vi "5x Lesen System ini.vi"(8 "Fehler (Eingang, kein Fehler)":errorcluster, 9 "Factorysettings":path, 11 "appended path":path) -> (0 "Fehler (Ausgang)":errorcluster, 2 "Sys Log Level":i32, 4 "Datenfluss (out)":bool)   [LabVIEW 2020, in "Konfig-Dateien.lvlib"]
uses:
  Konfig-Dateien.lvlib
  SysLog/SysLog Interface cRIO.ctl
  <vilib>/Utility/config.llb/Read Key (I32).vi
  <vilib>/Utility/config.llb/NI_LVConfig.lvlib
  SysLog/SysLog_cRIO.lvlib
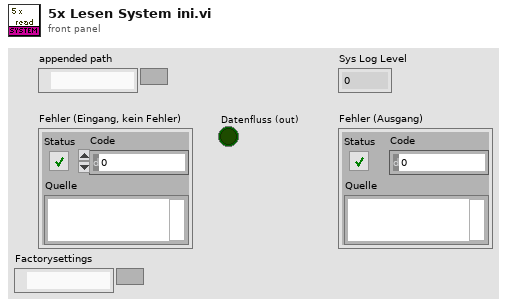
[diagram p1: front panel]
types:
  T1 = typedef "NI_LVConfig.lvlib/Config Data RefNum.ctl" = refnum<k1>
  T2 = typedef "SysLog_cRIO.lvlib/SysLog Interface cRIO.ctl" = cluster{"FehlermeldungsCode":i32, "ErfolgsmeldungsCode":i32, "ParameterListenString":string, "intern":bool}
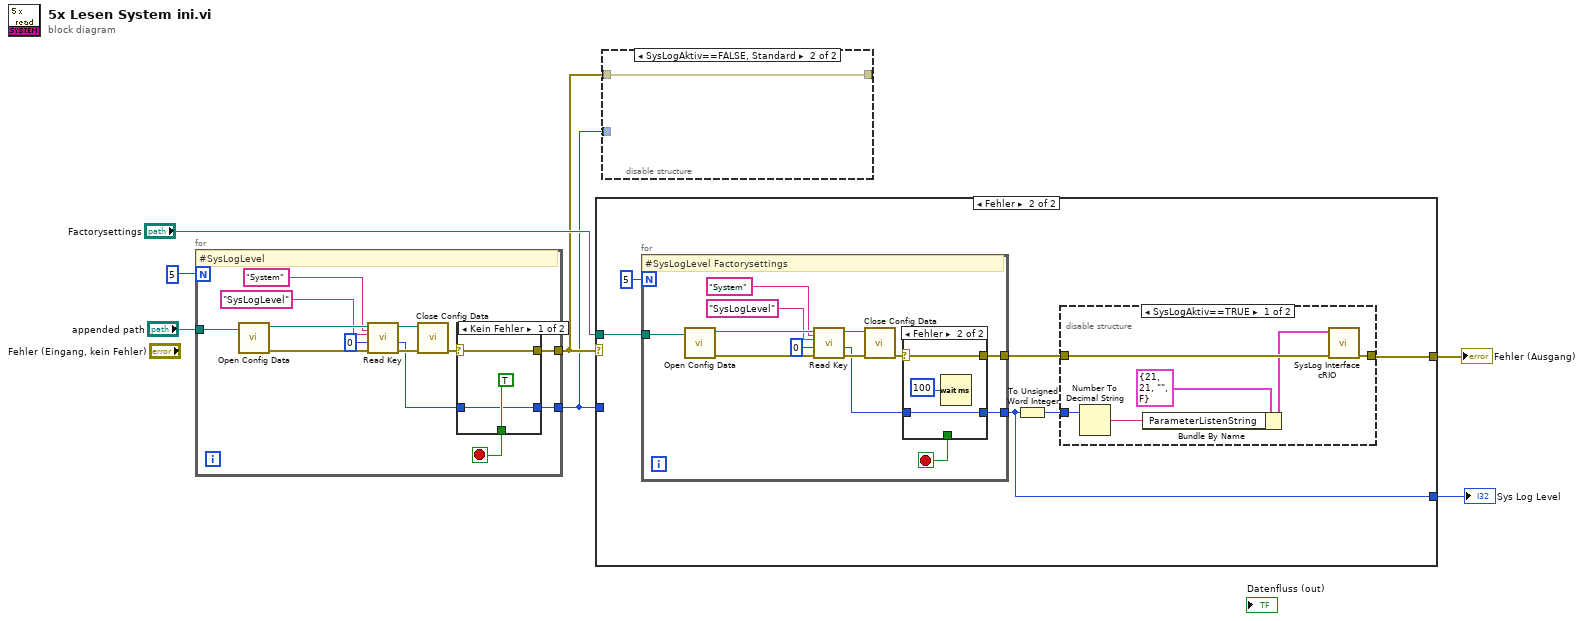
[diagram p0: block diagram]
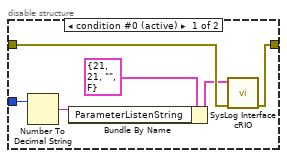
[diagram p2: hidden frame]
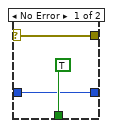
[diagram p5: hidden frame]
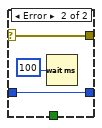
[diagram p6: hidden frame]
diagram:
  n1 = for {
    N: 5 -> [_]
    tunnel: "appended path" -> [w17]
    tunnel: [w11] -> w1
    tunnel: [w8] -> w2
    stop <- w20 stop-if-true
    # "#SysLogLevel"
    n2 = call <vilib>:"Open Config Data.vi"("configuration file path"=w17) -> ("error out"=w18:errorcluster, "refnum"=w19:T1)  [unwired: 8 in, 1 out]
    n3 = call-poly <vilib>:"Read Key.vi"("section"="System", "error in (no error)"=w18, "default value"=u32 0, "key"="SysLogLevel", "refnum"=w19) -> ("error out"=w14:errorcluster, "value"=w10:i32, "refnum out"=w13:T1)  [unwired: 3 in, 1 out]
    n4 = call <vilib>:"Close Config Data.vi"("error in (no error)"=w14, "refnum"=w13) -> ("error out"=w16:errorcluster)  [unwired: 8 in, 1 out]
    n5 = case shown="Kein Fehler" w16 {
      selector: w16 -> [w22 w26]
      tunnel: [TRUE _] -> w20
      tunnel: [w22 w26] -> w8
      tunnel: [w21 w25] -> w11
      tunnel: w10 -> [w21 w25]
      frame No Error {
      }
      frame Error {
        n6 = Wait (ms)(milliseconds to wait=u32 100 ("Zu wartende ms")) -> ()  [unwired: 1 out]
      }
    }
  }
  n7 = case shown="Fehler" w2 {
    selector: w2 -> [w27 _]
    tunnel: "Factorysettings" -> [_ w33]
    tunnel: [w28 w31] -> w3
    tunnel: w1 -> [w28 _]
    tunnel: [w27 w32] -> w4
    frame No Error {
    }
    frame Error {
      n8 = for {
        N: 5 -> [_]
        tunnel: w33 -> [w51]
        tunnel: [w45] -> w31
        tunnel: [w42] -> w29
        stop <- w54 stop-if-true
        # "#SysLogLevel Factorysettings"
        n9 = call <vilib>:"Open Config Data.vi"("configuration file path"=w51) -> ("error out"=w52:errorcluster, "refnum"=w53:T1)  [unwired: 8 in, 1 out]
        n10 = call-poly <vilib>:"Read Key.vi"("section"="System", "error in (no error)"=w52, "default value"=u32 0, "key"="SysLogLevel", "refnum"=w53) -> ("error out"=w48:errorcluster, "value"=w44:i32, "refnum out"=w47:T1)  [unwired: 3 in, 1 out]
        n11 = call <vilib>:"Close Config Data.vi"("error in (no error)"=w48, "refnum"=w47) -> ("error out"=w50:errorcluster)  [unwired: 8 in, 1 out]
        n12 = case shown="Fehler" w50 {
          selector: w50 -> [w56 w60]
          tunnel: [TRUE _] -> w54
          tunnel: [w56 w60] -> w42
          tunnel: [w55 w59] -> w45
          tunnel: w44 -> [w55 w59]
          frame No Error {
          }
          frame Error {
            n13 = Wait (ms)(milliseconds to wait=u32 100 ("Zu wartende ms")) -> ()  [unwired: 1 out]
          }
        }
      }
      n14 = To Unsigned Word Integer(number=w31) -> (unsigned 16bit integer=w30:u16)
      n15 = disable-structure shown="SysLogAktiv==TRUE" {
        disable-tunnel: [w40 w41] -> w32
        disable-tunnel: w29 -> [w39 w41]
        disable-tunnel: w30 -> [w35 _]
        frame condition #0 (active) {
          n16 = Number To Decimal String(number=w35) -> (decimal integer string=w36:string)  [unwired: 1 in]
          n17 = Bundle By Name(cluster=T2 {"FehlermeldungsCode"=21, "ErfolgsmeldungsCode"=21, "ParameterListenString"="", "intern"=FALSE} ("Cluster (in)"), "ParameterListenString"=w36) -> (w38:T2)
          n18 = call "SysLog Interface cRIO.vi"("Fehler (in)"=w39, "Cluster (in)"=w38) -> ("Fehler (Ausgang)"=w40:errorcluster)  [unwired: 9 in]
        }
        frame condition #1 {
        }
      }
    }
  }
  "Fehler (Ausgang)" <- w4
  "Sys Log Level" <- w3
  n19 = disable-structure shown="SysLogAktiv==FALSE, Standard" {
    disable-tunnel: [w66 w67] -> _
    disable-tunnel: w2 -> [w65 w67]
    disable-tunnel: w1 -> [w61 _]
    frame condition #0 (active) {
      n20 = Number To Decimal String(number=w61) -> (decimal integer string=w62:string)  [unwired: 1 in]
      n21 = Bundle By Name(cluster=T2 {"FehlermeldungsCode"=21, "ErfolgsmeldungsCode"=21, "ParameterListenString"="", "intern"=FALSE} ("Cluster (in)"), "ParameterListenString"=w62) -> (w64:T2)
      n22 = call "SysLog Interface cRIO.vi"("Fehler (in)"=w65, "Cluster (in)"=w64) -> ("Fehler (Ausgang)"=w66:errorcluster)  [unwired: 9 in]
    }
    frame condition #1 {
    }
  }
